vi "Initialize.vi"(8 "error in (no error)":errorcluster, 9 "Reset (True)":bool=TRUE, 10 "ID Query (True)":bool=TRUE, 11 "VISA resource name":refnum<visa-resource-name>) -> (0 "error out":errorcluster, 2 "idn string":string, 3 "VISA resource name out":refnum<visa-resource-name>)   [LabVIEW 2018, in "AWG.lvlib" / "Tektronix AFG 3000 Series.lvlib"]
doc: "Establishes communication with the instrument and optionally performs an instrument identification query and/or an instrument reset. It also places the instrument in a default state needed for other instrument driver operations. Therefore, call this VI before calling other instrument driver VIs for this instrument. Generally, you need to call the <B>Initialize VI</B> only once at the beginning of an application."
uses:
  Tektronix AFG 3000 Series.lvlib
panel:
  # "(c) 2006-2013 National Instruments.  ALL RIGHTS RESERVED."
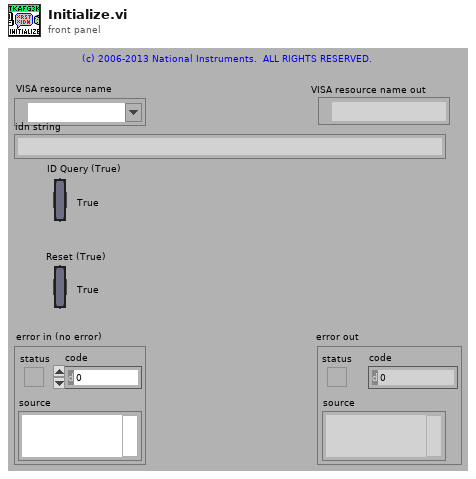
[diagram p1: front panel]
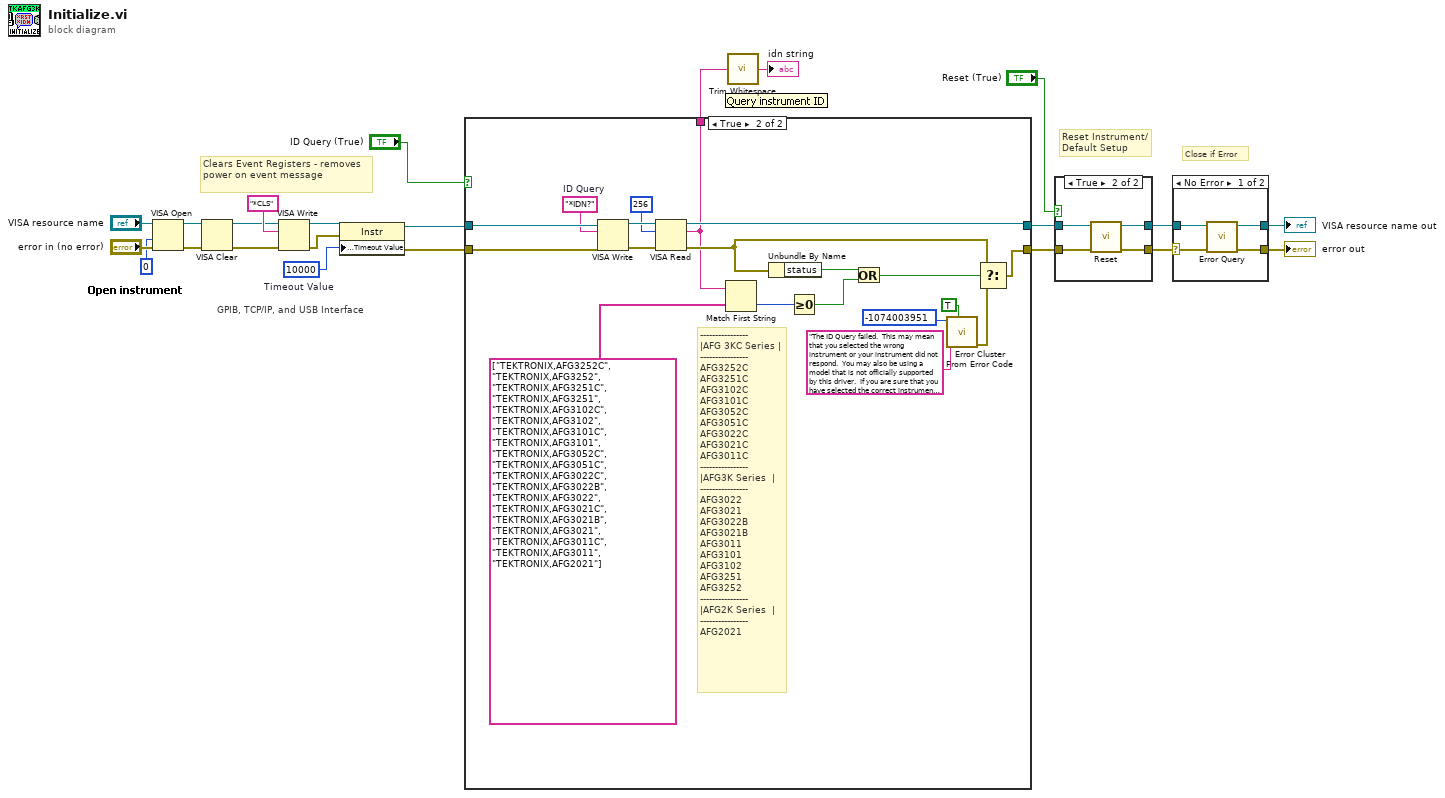
[diagram p0: block diagram]
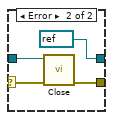
[diagram p2: hidden frame]
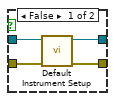
[diagram p3: hidden frame]
diagram:
  w8 = u32 10000  # Timeout Value
  # "Clears Event Registers - removes power on event message"
  # "GPIB, TCP/IP, and USB Interface"
  # "Close if Error"
  # "Reset Instrument/\nDefault Setup"
  n1 = VISA Open(access mode=u32 0, error in (no error)="error in (no error)", VISA resource name="VISA resource name") -> (VISA resource name=w18:refnum<visa-resource-name>, error out=w17:errorcluster)  [unwired: 2 in]
  n2 = VISA Clear(VISA resource name=w18, error in (no error)=w17) -> (VISA resource name out=w6:refnum<visa-resource-name>, error out=w5:errorcluster)
  n3 = VISA Write(VISA resource name=w6, write buffer="*CLS", error in (no error)=w5) -> (VISA resource name out=w4:refnum<visa-resource-name>, error out=w3:errorcluster)  [unwired: 1 out]
  n4 = property class="Instr"(reference=w4, error in=w3, "General Settings:Timeout Value"=w8) -> (reference out=w10:refnum<visa-resource-name>, error out=w9:errorcluster)
  n5 = case shown="True" "ID Query (True)" {
    tunnel: [w24 w33] -> w11
    tunnel: [w25 w42] -> w12
    tunnel: w10 -> [w25 w43]
    tunnel: w9 -> [w24 w44]
    tunnel: [_ w26] -> w2
    frame False {
    }
    frame True {
      w38 = "*IDN?"  # ID Query
      # "----------------\n|AFG 3KC Series |\n----------------\nAFG3252C\nAFG3251C\nAFG3102C\nAFG3101C\nAFG3052C\nAFG3051C\nAFG3022C\nAFG3021C\nAFG3011C\n----------------\n|AFG3K Series  |\n----------------\nAFG3022\nAFG3021\nAFG3022B\nAFG3021B\nAFG3011\nAFG3101\nAFG3102\nAFG3251\nAFG3252\n----------------\n|AFG2K Series  |\n----------------\nAFG2021"
      n6 = VISA Write(VISA resource name=w43, write buffer=w38, error in (no error)=w44) -> (VISA resource name out=w41:refnum<visa-resource-name>, error out=w40:errorcluster)  [unwired: 1 out]
      n7 = VISA Read(VISA resource name=w41, byte count=u32 256, error in (no error)=w40) -> (VISA resource name out=w42:refnum<visa-resource-name>, read buffer=w26:string, error out=w37:errorcluster)  [unwired: 1 out]
      n8 = Match First String(2:string[] ["TEKTRONIX,AFG3252C", "TEKTRONIX,AFG3252", "TEKTRONIX,AFG3251C", "TEKTRONIX,AFG3251", "TEKTRONIX,AFG3102C", "TEKTRONIX,AFG3102", "TEKTRONIX,AFG3101C", "TEKTRONIX,AFG3101", "TEKTRONIX,AFG3052C", "TEKTRONIX,AFG3051C", "TEKTRONIX,AFG3022C", "TEKTRONIX,AFG3022B", "TEKTRONIX,AFG3022", "TEKTRONIX,AFG3021C", "TEKTRONIX,AFG3021B", "TEKTRONIX,AFG3021", "TEKTRONIX,AFG3011C", "TEKTRONIX,AFG3011", "TEKTRONIX,AFG2021"] ("reversed array"), 3:w26) -> (0:w28:i32)  [unwired: 1 out]
      n9 = Unbundle By Name(w37) -> ("status"=w36:bool)
      n10 = Greater Or Equal To 0?(x=w28) -> (x >= 0?=w35:bool)
      n11 = Or(x=w36, y=w35) -> (x .or. y?=w34:bool)
      n12 = call <vilib>:"Error Cluster From Error Code.vi"("show call chain? (False)"=TRUE, "error message (\"\")"="The ID Query failed.  This may mean that you selected the wrong instrument or your instrument did not respond.  You may also be using a model that is not officially supported by this driver.  If you are sure that you have selected the correct instrument and it is responding, try disabling the ID Query." ("Source (VI Name)"), "error code (0)"=-1074003951 ("Code")) -> ("error out"=w29:errorcluster)  [unwired: 6 in]
      n13 = Select(t=w37, s=w34, f=w29) -> (s? t:f=w33:errorcluster)
    }
  }
  n14 = call <vilib>:"Trim Whitespace.vi"("string"=w2) -> ("trimmed string"=→"idn string":string)  [unwired: 1 in]
  n15 = case shown="True" "Reset (True)" {
    tunnel: [w47 w52] -> w13
    tunnel: w12 -> [w48 w50]
    tunnel: [w46 w51] -> w14
    tunnel: w11 -> [w45 w49]
    frame False {
      n16 = call "Default Instrument Setup.vi"("error in (no error)"=w45, "VISA resource name"=w48) -> ("error out"=w47:errorcluster, "VISA resource name out"=w46:refnum<visa-resource-name>)  [unwired: 8 in]
    }
    frame True {
      n17 = call "Reset.vi"("error in (no error)"=w49, "VISA resource name"=w50) -> ("error out"=w52:errorcluster, "VISA resource name out"=w51:refnum<visa-resource-name>)  [unwired: 8 in]
    }
  }
  n18 = case shown="No Error" w13 {
    selector: w13 -> [w54 w58]
    tunnel: w14 -> [w53 w59]
    tunnel: [w56 refnum<visa-resource-name> refnum ("VISA resource name out")] -> w16
    tunnel: [w55 w60] -> w15
    frame No Error {
      n19 = call "Error Query.vi"("error in (no error)"=w54, "VISA resource name"=w53) -> ("error out"=w55:errorcluster, "VISA resource name out"=w56:refnum<visa-resource-name>)  [unwired: 6 in, 2 out]
    }
    frame Error {
      n20 = call "Close.vi"("error in (no error)"=w58, "VISA resource name"=w59) -> ("error out"=w60:errorcluster)  [unwired: 9 in]
    }
  }
  "VISA resource name out" <- w16
  "error out" <- w15
